vi "ControlerVibrationManager.vi"(9 "Rumble Intensity":sgl=2.0, 10 "Setpoint Duration":dbl) -> ()   [LabVIEW 2014]
uses:
  <vilib>/Rock Robotics/WPI/Joystick/WPI_JoystickGetSetRefNum.vi
  Robot Global Data.vi
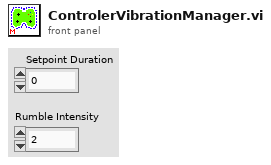
[diagram p1: front panel]
types:
  T1 = typedef "WPI_JoystickDevRef.ctl" = cluster{"Device":T2}
  T2 = typedef "WPI_JoystickDeviceEnum.ctl" = enum16{"USB 0", "USB 1", "USB 2", "USB 3", "USB 4", "USB 5"}
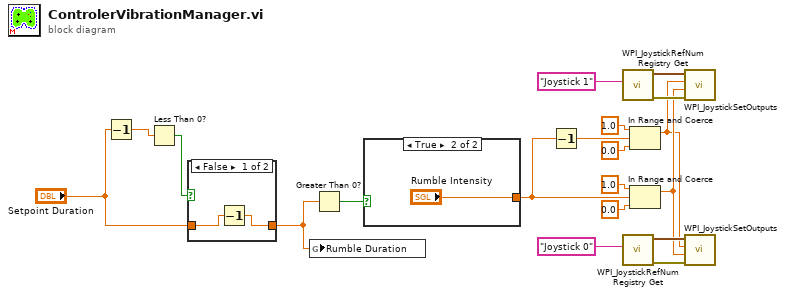
[diagram p0: block diagram]
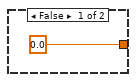
[diagram p3: hidden frame]
diagram:
  n1 = Decrement(x="Setpoint Duration") -> (x-1=w5:dbl)
  n2 = Less Than 0?(x=w5) -> (x < 0?=w4:bool)
  n3 = case shown="False" w4 {
    tunnel: "Setpoint Duration" -> [w21 w22]
    tunnel: [w20 w22] -> w1
    frame False {
      n4 = Decrement(x=w21) -> (x-1=w20:dbl)
    }
    frame True {
    }
  }
  n5 = global write "Robot Global Data.vi" "Rumble Duration"(w1) -> ()
  n6 = Greater Than 0?(x=w1) -> (x > 0?=w2:bool)
  n7 = case shown="True" w2 {
    tunnel: [sgl 0.0 ("Left Rumble") "Rumble Intensity"] -> w10
    frame False {
    }
    frame True {
    }
  }
  n8 = Decrement(x=w10) -> (x-1=w7:sgl)
  n9 = call <vilib>:"WPI_JoystickRefNum Registry Get.vi"("refnum name"="Joystick 1") -> ("error out"=w17:errorcluster, "JoystickDevRef"=w18:T1)  [unwired: 9 in]
  n10 = call <vilib>:"WPI_JoystickRefNum Registry Get.vi"("refnum name"="Joystick 0") -> ("error out"=w14:errorcluster, "JoystickDevRef"=w15:T1)  [unwired: 9 in]
  n11 = In Range and Coerce(upper limit=sgl 1.0, x=w7, lower limit=sgl 0.0) -> (coerced(x)=w6:sgl)  [unwired: 1 out]
  n12 = In Range and Coerce(upper limit=sgl 1.0, x=w10, lower limit=sgl 0.0) -> (coerced(x)=w13:sgl)  [unwired: 1 out]
  n13 = call <vilib>:"WPI_JoystickSetOutputs.vi"("error in (no error)"=w17, "Right Rumble"=w13, "Left Rumble"=w6, "JoystickDevRef"=w18) -> ()  [unwired: 6 in, 2 out]
  n14 = call <vilib>:"WPI_JoystickSetOutputs.vi"("error in (no error)"=w14, "Right Rumble"=w13, "Left Rumble"=w6, "JoystickDevRef"=w15) -> ()  [unwired: 6 in, 2 out]
